vi "Omniax_mDrive_GNDMonitor.vi"() -> ()   [LabVIEW 2015]
uses:
  Omniax_mDrive_GNDGlobal.vi
panel:
  in  "stop":bool
  out "NC":bool
  in  "Open?":bool
  out "sum":dbl
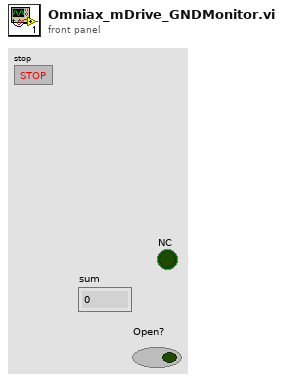
[diagram p1: front panel]
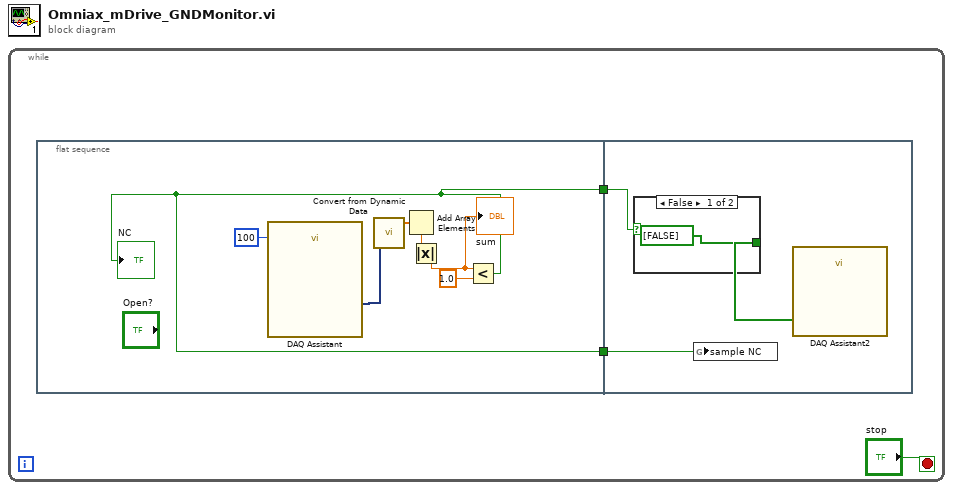
[diagram p0: block diagram]
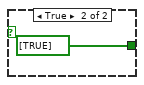
[diagram p2: hidden frame]
diagram:
  n1 = while {
    stop <- "stop" stop-if-true
    n2 = flat-sequence {
      tunnel: [w4] -> w3
      tunnel: [w4] -> w1
      tunnel: w3 -> [w13]
      tunnel: w1 -> [w11]
      frame #0 {
        n3 = call "DAQ Assistant"("number of samples"=100) -> ("data"=w9:dynamicdata)  [unwired: 16 in, 2 out]
        n4 = call "Convert from Dynamic Data"("Dynamic Data Type"=w9) -> ("Array"=w8:dbl[])  [unwired: 3 in]
        n5 = Add Array Elements(numeric array=w8) -> (sum=w7:dbl)
        n6 = Absolute Value(x=w7) -> (abs(x)=w5:dbl)
        "sum" <- w5
        n7 = Less?(x=w5, y=1.0) -> (x < y?=w4:bool)
        "NC" <- w4
      }
      frame #1 {
        n8 = case shown="False" w13 {
          tunnel: [bool[] [FALSE] ("data") bool[] [TRUE] ("data")] -> w12
          frame False {
          }
          frame True {
          }
        }
        n9 = global write "Omniax_mDrive_GNDGlobal.vi" "sample NC"(w11) -> ()
        n10 = call "DAQ Assistant2"("data"=w12) -> ()  [unwired: 17 in, 2 out]
      }
    }
  }
